vi "test_GetItemInfosFromProjectFile_TargetsDifferentCompilersSolution.vi"() -> (3 "Pass?":bool)   [LabVIEW 2019, in "Tests.SolutionBuilder.lvlib"]
uses:
  Tests.SolutionBuilder.lvlib
  SolutionBuilder/SolutionBuilder.lvclass
  SolutionBuilder/ProjectItem/ProjectItem.lvclass
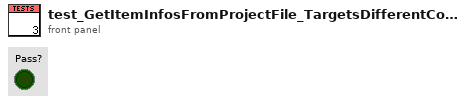
[diagram p1: front panel]
types:
  T1 = typedef "SolutionBuilder.lvlib/SolutionBuilder.lvclass/ProjectItemMap.ctl" = map{path, refnum<class "ProjectItem.lvclass">[]}
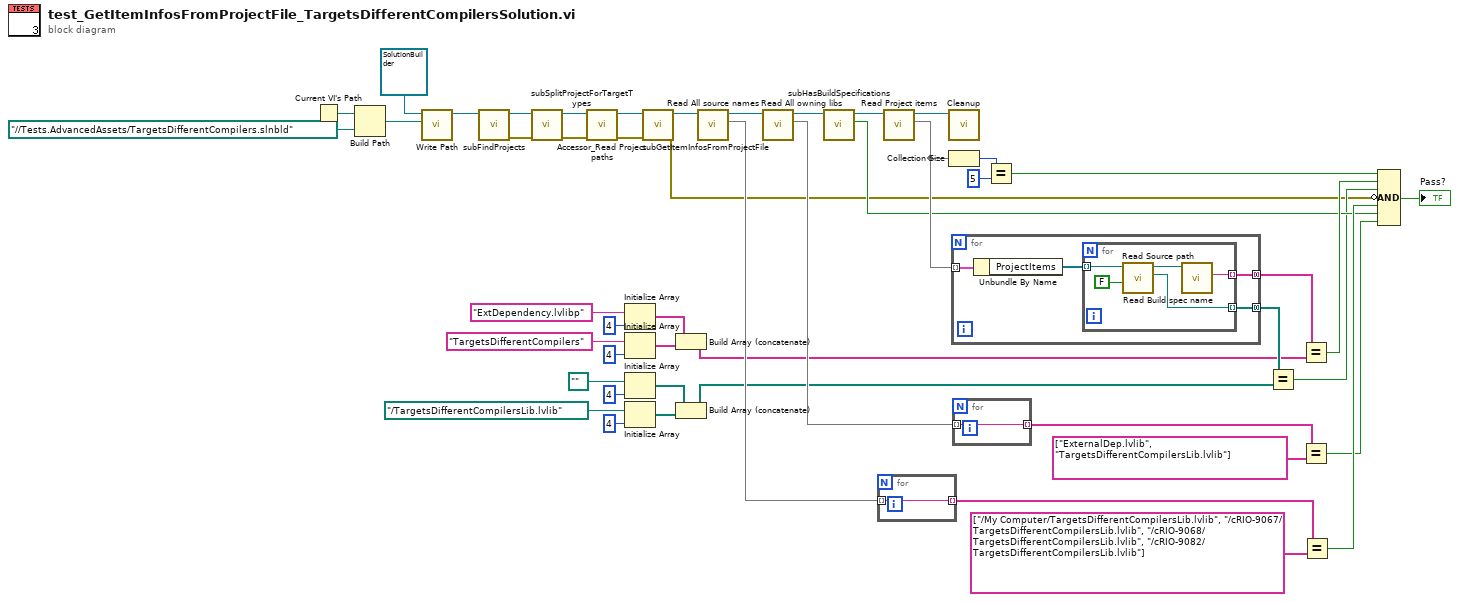
[diagram p0: block diagram]
diagram:
  n1 = Current VI's Path() -> (path=w47:path)
  n2 = Build Path(base path=w47, name or relative path=path "../../Tests.AdvancedAssets/TargetsDifferentCompilers.slnbld" ("Path")) -> (appended path=w45:path)
  n3 = call "Write Path.vi"("Path"=w45, "SolutionBuilder in"=refnum<class "SolutionBuilder.lvclass"> refnum) -> ("SolutionBuilder out"=w48:refnum<class "SolutionBuilder.lvclass">)  [unwired: 9 in]
  n4 = call "subFindProjects.vi"("SolutionBuilder in"=w48) -> ("error out"=w4:errorcluster, "SolutionBuilder out"=w5:refnum<class "SolutionBuilder.lvclass">)  [unwired: 9 in]
  n5 = call "subSplitProjectForTargetTypes.vi"("error in (no error)"=w4, "SolutionBuilder in"=w5) -> ("error out"=w8:errorcluster, "SolutionBuilder out"=w9:refnum<class "SolutionBuilder.lvclass">)  [unwired: 8 in]
  n6 = call "Accessor_Read Project paths.vi"("error in (no error)"=w8, "SolutionBuilder in"=w9) -> ("error out"=w6:errorcluster, "SolutionBuilder out"=w7:refnum<class "SolutionBuilder.lvclass">)  [unwired: 7 in, 1 out]
  n7 = Initialize Array("ExtDependency.lvlibp" ("Build spec name"), 4 ("dimension size")) -> (w19:string[])
  n8 = Initialize Array("TargetsDifferentCompilers" ("Build spec name"), 4 ("dimension size")) -> (w1:string[])
  n9 = Initialize Array(path "" ("Source path"), 4 ("dimension size")) -> (w17:path[])
  n10 = Initialize Array(path "../TargetsDifferentCompilersLib.lvlib" ("Source path"), 4 ("dimension size")) -> (w2:path[])
  n11 = call "subGetItemInfosFromProjectFile.vi"("error in (no error)"=w6, "SolutionBuilder in"=w7) -> ("error out"=w24:errorcluster, "SolutionBuilder out"=w42:refnum<class "SolutionBuilder.lvclass">)  [unwired: 8 in]
  n12 = Build Array (concatenate)(w19, w1) -> (w18:string[])
  n13 = Build Array (concatenate)(w17, w2) -> (w12:path[])
  n14 = call "Read All source names.vi"("SolutionBuilder in"=w42) -> ("All source names"=w38:set{string}, "SolutionBuilder out"=w30:refnum<class "SolutionBuilder.lvclass">)  [unwired: 9 in]
  n15 = call "Read All owning libs.vi"("SolutionBuilder in"=w30) -> ("All owning libs"=w28:set{string}, "SolutionBuilder out"=w29:refnum<class "SolutionBuilder.lvclass">)  [unwired: 9 in]
  n16 = call "subHasBuildSpecifications.vi"("SolutionBuilder in"=w29) -> ("Has specs?"=w35:bool, "SolutionBuilder out"=w36:refnum<class "SolutionBuilder.lvclass">)  [unwired: 8 in, 1 out]
  n17 = for {
    tunnel: w38 -> [w50] mode=indexing
    tunnel: [w50] -> w33 mode=indexing
  }
  n18 = call "Read Project items.vi"("SolutionBuilder in"=w36) -> ("Project items"=w41:T1, "SolutionBuilder out"=w10:refnum<class "SolutionBuilder.lvclass">)  [unwired: 9 in]
  n19 = call "Cleanup.vi"("SolutionBuilder in"=w10) -> ()  [unwired: 9 in, 2 out]
  n20 = Collection Size(1:w41) -> (0:w44:i32)
  n21 = for {
    tunnel: w41 -> [w54] mode=indexing
    tunnel: [w53] -> w34 mode=concatenating
    tunnel: [w51] -> w32 mode=concatenating
    n22 = Unbundle By Name(w54) -> ("ProjectItems"=w52:refnum<class "ProjectItem.lvclass">[])
    n23 = for {
      tunnel: w52 -> [w57] mode=indexing
      tunnel: [w59] -> w53 mode=indexing
      tunnel: [w56] -> w51 mode=indexing
      n24 = call "Read Source path.vi"("Force abs path? (T)"=FALSE, "ProjectItem in"=w57) -> ("Source path"=w56:path, "ProjectItem out"=w58:refnum<class "ProjectItem.lvclass">)  [unwired: 8 in]
      n25 = call "Read Build spec name.vi"("ProjectItem in"=w58) -> ("Build spec name"=w59:string)  [unwired: 9 in, 1 out]
    }
  }
  n26 = for {
    tunnel: w28 -> [w60] mode=indexing
    tunnel: [w60] -> w27 mode=indexing
  }
  n27 = Equal?(x=w44, y=5) -> (x = y?=w40:bool)
  n28 = Equal?(x=w32, y=w12) -> (x = y?=w31:bool)
  n29 = Equal?(x=w34, y=w18) -> (x = y?=w39:bool)
  n30 = Equal?(x=w27, y=string[] ["ExternalDep.lvlib", "TargetsDifferentCompilersLib.lvlib"] ("Array")) -> (x = y?=w25:bool)
  n31 = Equal?(x=w33, y=string[] ["/My Computer/TargetsDifferentCompilersLib.lvlib", "/cRIO-9067/TargetsDifferentCompilersLib.lvlib", "/cRIO-9068/TargetsDifferentCompilersLib.lvlib", "/cRIO-9082/TargetsDifferentCompilersLib.lvlib"] ("Array")) -> (x = y?=w37:bool)
  n32 = Compound Arithmetic op=AND(w40, w39, w31, invert w24, w37, w35, w25) -> (→"Pass?":bool)
